vi "tm3samp_dualsync.vi"() -> ()   [LabVIEW 2011]
panel:
  out "Camera Model":string
  out "Image 1":u16[][](graph) caption="Image"
  in  "capture":bool
  out "Image 2":u16[][](graph) caption="Image"
  in  "Quit":bool
  out "Error Out":errorcluster
  # "This is an example of one way\nto synchronize two of the same\nmodel cameras."
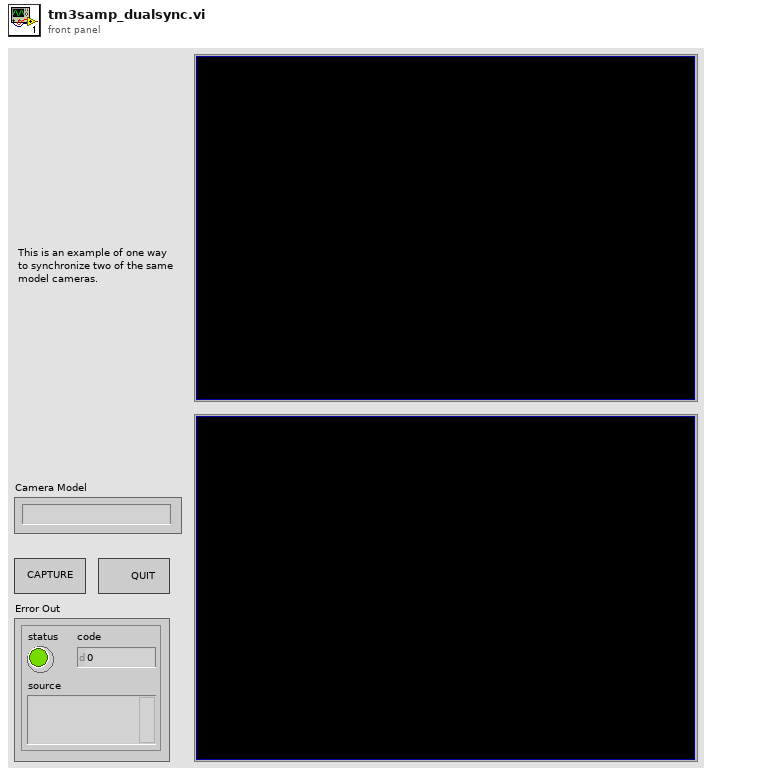
[diagram p1: front panel]
types:
  T1 = cluster{"width":u32, "height":u32, "datatype":u32}
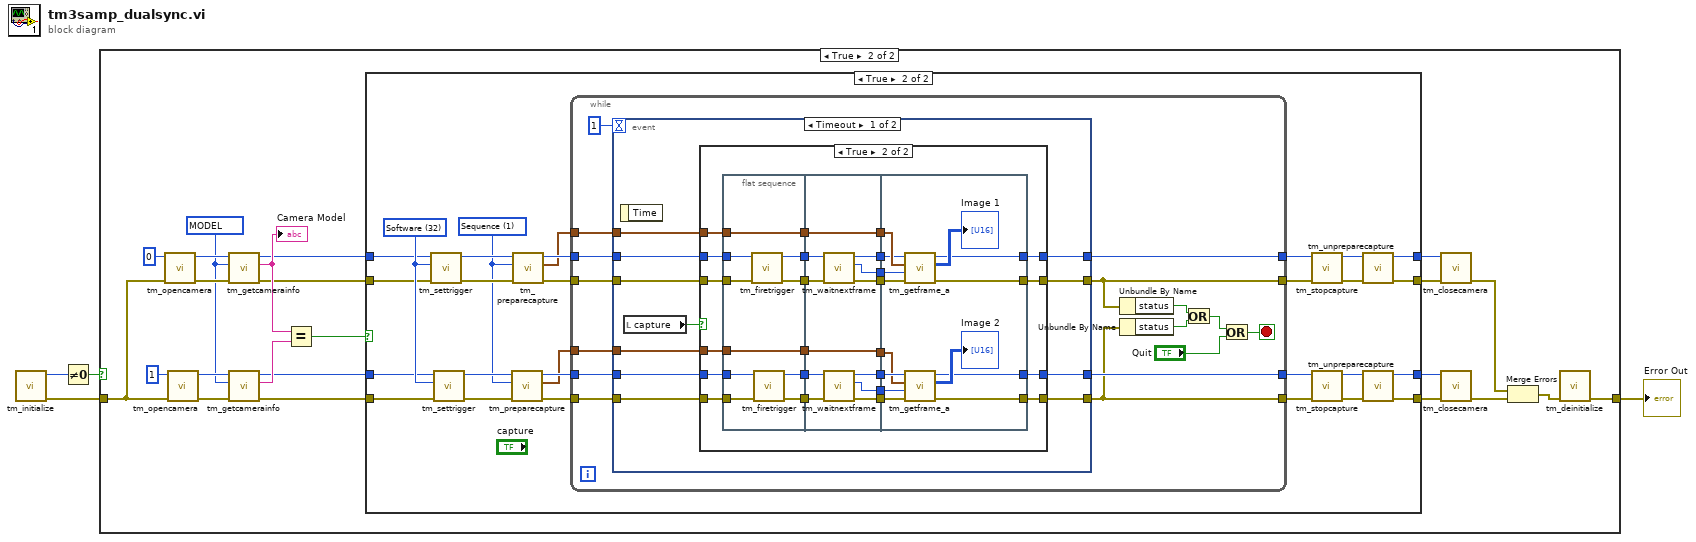
[diagram p0: block diagram]
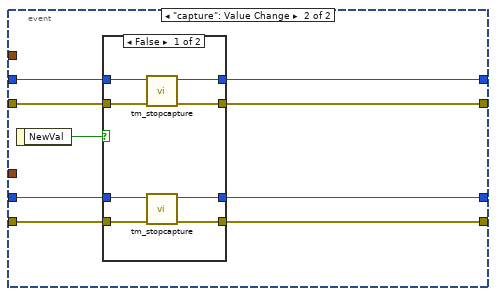
[diagram p5: hidden frame]
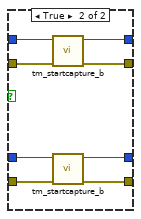
[diagram p6: hidden frame]
diagram:
  n1 = call <userlib>:"tm_initialize.vi"() -> ("error out"=w1:errorcluster, "Number Of Cameras"=w2:u32)  [unwired: 10 in]
  n2 = Not Equal To 0?(x=w2) -> (x != 0?=w4:bool)
  n3 = case shown="True" w4 {
    tunnel: w1 -> [w5 w25]
    tunnel: [w5 w27] -> w3
    frame False {
    }
    frame True {
      w17 = u32 67109124 items=["BUS"=67109121, "CAMERA ID"=67109122, "VENDOR"=67109123, "MODEL"=67109124, "CAMERA VERSION"=67109125, "DRIVER VERSION"=67109126, "MODULE VERSIOIN"=67109127, "DCAMAPI VERSION"=67109128] ("Info ID")
      n4 = call <userlib>:"tm_opencamera.vi"("error in (no error)"=w25, "Camera Index"=u32 0) -> ("error out"=w20:errorcluster, "Handle out"=w21:u32)  [unwired: 8 in]
      n5 = call <userlib>:"tm_opencamera.vi"("error in (no error)"=w25, "Camera Index"=u32 1) -> ("error out"=w18:errorcluster, "Handle out"=w19:u32)  [unwired: 8 in]
      n6 = call <userlib>:"tm_getcamerainfo.vi"("error in (no error)"=w20, "Info ID"=w17, "Handle in"=w21) -> ("error out"=w11:errorcluster, "String"=w15:string, "Handle out"=w10:u32)  [unwired: 6 in]
      "Camera Model" <- w15
      n7 = call <userlib>:"tm_getcamerainfo.vi"("error in (no error)"=w18, "Info ID"=w17, "Handle in"=w19) -> ("error out"=w12:errorcluster, "String"=w16:string, "Handle out"=w13:u32)  [unwired: 6 in]
      n8 = Equal?(x=w15, y=w16) -> (x = y?=w14:bool)
      n9 = case shown="True" w14 {
        tunnel: w13 -> [w32 w38]
        tunnel: w12 -> [w31 w37]
        tunnel: w11 -> [w30 w33]
        tunnel: w10 -> [w29 w34]
        tunnel: [w32 w40] -> w9
        tunnel: [w31 w39] -> w8
        tunnel: [w30 w35] -> w7
        tunnel: [w29 w36] -> w6
        frame False {
        }
        frame True {
          w41 = u32 32 items=["Internal"=1, "External Edge"=2, "External Level"=4, "Software"=32, "Fast Repetition"=64, "TDI"=128, "Trigger Start"=512, "Sync Readout"=1024] ("Trigger Mode")
          w42 = 1 items=["Snap", "Sequence"] ("Capture mode")
          n10 = call <userlib>:"tm_settrigger.vi"("error in (no error)"=w33, "Trigger Mode"=w41, "Handle in"=w34) -> ("error out"=w50:errorcluster, "Handle out"=w51:u32)  [unwired: 7 in]
          n11 = call <userlib>:"tm_settrigger.vi"("error in (no error)"=w37, "Trigger Mode"=w41, "Handle in"=w38) -> ("error out"=w52:errorcluster, "Handle out"=w53:u32)  [unwired: 7 in]
          n12 = call <userlib>:"tm_preparecapture.vi"("error in (no error)"=w52, "Capture mode"=w42, "Handle in"=w53) -> ("error out"=w59:errorcluster, "Buffer"=w58:T1, "Handle out"=w60:u32)  [unwired: 5 in, 1 out]
          n13 = call <userlib>:"tm_preparecapture.vi"("error in (no error)"=w50, "Capture mode"=w42, "Handle in"=w51) -> ("error out"=w48:errorcluster, "Buffer"=w47:T1, "Handle out"=w49:u32)  [unwired: 5 in, 1 out]
          n14 = while {
            tunnel: [w74] -> w57
            tunnel: [w66] -> w56
            tunnel: w60 -> [w76]
            tunnel: w59 -> [w75]
            tunnel: w58 -> [w73]
            tunnel: w49 -> [w70]
            tunnel: w48 -> [w69]
            tunnel: w47 -> [w68]
            tunnel: [w65] -> w43
            tunnel: [w67] -> w44
            stop <- w63 stop-if-true
            n15 = event shown="[0] Timeout" {
              selector: _ -> [_ _]
              dyn-events: _ -> [_ _]
              timeout: 1 -> [_ _]
              tunnel: w76 -> [w82 w159]
              tunnel: w75 -> [w81 w158]
              tunnel: [w78 w157] -> w74
              tunnel: [w77 w156] -> w66
              tunnel: w73 -> [w83 _]
              tunnel: w70 -> [w85 w155]
              tunnel: w68 -> [w86 _]
              tunnel: w69 -> [w84 w154]
              tunnel: [w79 w152] -> w67
              tunnel: [w80 w153] -> w65
              event Timeout {
                n16 = event-data() -> ()  [unwired: 1 in, 1 out]
                n17 = local read "capture"() -> (w87:bool)
                n18 = case shown="True" w87 {
                  tunnel: w86 -> [_ w103]
                  tunnel: w85 -> [w91 w102]
                  tunnel: w84 -> [w90 w101]
                  tunnel: w83 -> [_ w100]
                  tunnel: w82 -> [w88 w99]
                  tunnel: w81 -> [w89 w98]
                  tunnel: [w90 w97] -> w80
                  tunnel: [w91 w96] -> w79
                  tunnel: [w88 w95] -> w78
                  tunnel: [w89 w94] -> w77
                  frame False {
                  }
                  frame True {
                    n19 = flat-sequence {
                      tunnel: w99 -> [w125]
                      tunnel: w98 -> [w124]
                      tunnel: [w123] -> w115
                      tunnel: [w122] -> w114
                      tunnel: w100 -> [w121]
                      tunnel: [w121] -> w113
                      tunnel: w103 -> [w120]
                      tunnel: [w120] -> w112
                      tunnel: w102 -> [w119]
                      tunnel: [w117] -> w111
                      tunnel: w101 -> [w118]
                      tunnel: [w116] -> w110
                      tunnel: w115 -> [w134]
                      tunnel: w114 -> [w135]
                      tunnel: w113 -> [w128]
                      tunnel: w112 -> [w133]
                      tunnel: w111 -> [w136]
                      tunnel: w110 -> [w137]
                      tunnel: [w133] -> w109
                      tunnel: [w132] -> w108
                      tunnel: [w131] -> w107
                      tunnel: [w130] -> w106
                      tunnel: [w129] -> w105
                      tunnel: [w128] -> w104
                      tunnel: [w126] -> w93
                      tunnel: [w127] -> w92
                      tunnel: w109 -> [w149]
                      tunnel: w108 -> [w147]
                      tunnel: w107 -> [w148]
                      tunnel: [w146] -> w96
                      tunnel: [w145] -> w97
                      tunnel: w106 -> [w144]
                      tunnel: w105 -> [w143]
                      tunnel: w104 -> [w142]
                      tunnel: [w141] -> w95
                      tunnel: [w140] -> w94
                      tunnel: w93 -> [w139]
                      tunnel: w92 -> [w138]
                      frame #0 {
                        n20 = call <userlib>:"tm_firetrigger.vi"("error in (no error)"=w118, "Handle in"=w119) -> ("error out"=w116:errorcluster, "Handle out"=w117:u32)  [unwired: 8 in]
                        n21 = call <userlib>:"tm_firetrigger.vi"("error in (no error)"=w124, "Handle in"=w125) -> ("error out"=w122:errorcluster, "Handle out"=w123:u32)  [unwired: 8 in]
                      }
                      frame #1 {
                        n22 = call <userlib>:"tm_waitnextframe.vi"("error in (no error)"=w137, "Handle in"=w136) -> ("error out"=w131:errorcluster, "Frame Index"=w126:i32, "Handle out"=w132:u32)  [unwired: 6 in, 1 out]
                        n23 = call <userlib>:"tm_waitnextframe.vi"("error in (no error)"=w135, "Handle in"=w134) -> ("error out"=w129:errorcluster, "Frame Index"=w127:i32, "Handle out"=w130:u32)  [unwired: 6 in, 1 out]
                      }
                      frame #2 {
                        n24 = call <userlib>:"tm_getframe_a.vi"("error in (no error)"=w148, "Frame Index"=w139, "Buffer"=w149, "Handle in"=w147) -> ("error out"=w145:errorcluster, "Data 16"=→"Image 1":u16[][], "Handle out"=w146:u32)  [unwired: 3 in, 2 out]
                        n25 = call <userlib>:"tm_getframe_a.vi"("error in (no error)"=w143, "Frame Index"=w138, "Buffer"=w142, "Handle in"=w144) -> ("error out"=w140:errorcluster, "Data 16"=→"Image 2":u16[][], "Handle out"=w141:u32)  [unwired: 3 in, 2 out]
                      }
                    }
                  }
                }
              }
              event "capture": Value Change {
                n26 = event-data() -> ("NewVal"=w160:bool)  [unwired: 1 in]
                n27 = case shown="False" w160 {
                  tunnel: w159 -> [w168 w176]
                  tunnel: w158 -> [w167 w175]
                  tunnel: [w166 w174] -> w157
                  tunnel: [w165 w173] -> w156
                  tunnel: w155 -> [w163 w172]
                  tunnel: w154 -> [w164 w171]
                  tunnel: [w162 w170] -> w152
                  tunnel: [w161 w169] -> w153
                  frame False {
                    n28 = call <userlib>:"tm_stopcapture.vi"("error in (no error)"=w164, "Handle in"=w163) -> ("error out"=w161:errorcluster, "Handle out"=w162:u32)  [unwired: 8 in]
                    n29 = call <userlib>:"tm_stopcapture.vi"("error in (no error)"=w167, "Handle in"=w168) -> ("error out"=w165:errorcluster, "Handle out"=w166:u32)  [unwired: 8 in]
                  }
                  frame True {
                    n30 = call <userlib>:"tm_startcapture_b.vi"("error in (no error)"=w171, "Handle in"=w172) -> ("error out"=w169:errorcluster, "Handle out"=w170:u32)  [unwired: 8 in]
                    n31 = call <userlib>:"tm_startcapture_b.vi"("error in (no error)"=w175, "Handle in"=w176) -> ("error out"=w173:errorcluster, "Handle out"=w174:u32)  [unwired: 8 in]
                  }
                }
              }
            }
            n32 = Unbundle By Name(w65) -> ("status"=w72:bool)
            n33 = Unbundle By Name(w66) -> ("status"=w64:bool)
            n34 = Or(x=w72, y=w64) -> (x .or. y?=w62:bool)
            n35 = Or(x=w62, y="Quit") -> (x .or. y?=w63:bool)
          }
          n36 = call <userlib>:"tm_stopcapture.vi"("error in (no error)"=w43, "Handle in"=w44) -> ("error out"=w45:errorcluster, "Handle out"=w46:u32)  [unwired: 8 in]
          n37 = call <userlib>:"tm_stopcapture.vi"("error in (no error)"=w56, "Handle in"=w57) -> ("error out"=w54:errorcluster, "Handle out"=w55:u32)  [unwired: 8 in]
          n38 = call <userlib>:"tm_unpreparecapture.vi"("error in (no error)"=w45, "Handle in"=w46) -> ("error out"=w35:errorcluster, "Handle out"=w36:u32)  [unwired: 8 in]
          n39 = call <userlib>:"tm_unpreparecapture.vi"("error in (no error)"=w54, "Handle in"=w55) -> ("error out"=w39:errorcluster, "Handle out"=w40:u32)  [unwired: 8 in]
        }
      }
      n40 = call <userlib>:"tm_closecamera.vi"("error in (no error)"=w7, "Handle in"=w6) -> ("error out"=w24:errorcluster)  [unwired: 9 in]
      n41 = call <userlib>:"tm_closecamera.vi"("error in (no error)"=w8, "Handle in"=w9) -> ("error out"=w23:errorcluster)  [unwired: 9 in]
      n42 = Merge Errors(w24, w23) -> (w22:errorcluster)
      n43 = call <userlib>:"tm_deinitialize.vi"("error in (no error)"=w22) -> ("error out"=w27:errorcluster)  [unwired: 10 in]
    }
  }
  "Error Out" <- w3
